vi "时间与数值的转换.vi"() -> ()   [LabVIEW 2020]
doc: "本VI是为《我和LabVIEW》一书编写的示例。\n关于本书的介绍请参考网页：\nhttp://ruanqizhen.spaces.live.com/blog/cns!5852D4F797C53FB6!4310.entry"
panel:
  out "时间标识":timestamp
  out "手工转换整数部分":u64
  out "手工转换小数部分":ext format="%#.6f"
  out "内部类型":cluster{u64, u64} {"?" format="%016x"; "?" format="%016x"}
  out "直接转换得到的秒数":dbl format="%.6f"
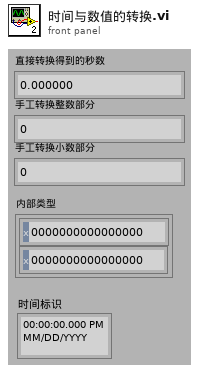
[diagram p1: front panel]
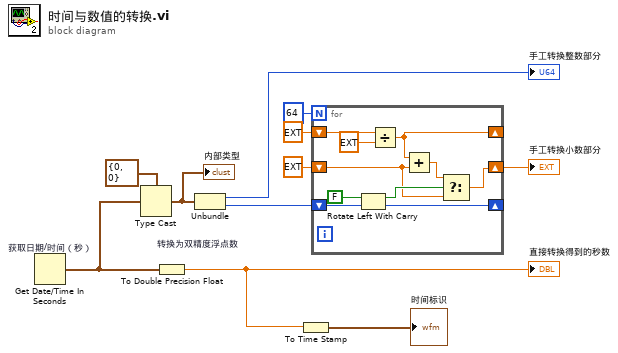
[diagram p0: block diagram]
diagram:
  n1 = Get Date/Time In Seconds "获取日期/时间（秒）"() -> (seconds since 1Jan1904=w11:timestamp)
  n2 = Type Cast(type=cluster{u64, u64} {0, 0}, x=w11) -> (*(type *) &x=w10:cluster{u64, u64})
  "内部类型" <- w10
  n3 = To Double Precision Float "转换为双精度浮点数"(number=w11) -> (double precision float=w2:dbl)
  "直接转换得到的秒数" <- w2
  n4 = Unbundle(w10) -> (→"手工转换整数部分":u64, w8:u64)
  n5 = To Time Stamp(1:w2) -> (0:→"时间标识":timestamp)
  n6 = for {
    N: 64 -> [_]
    shift-right: [w20] -> _
    shift-left: w8 -> [w21]
    shift-right: [w16] -> _
    shift-left: ext 1.0 -> [w19]
    shift-right: [w13] -> w6
    shift-left: ext 0.0 ("扩展精度浮点数") -> [w14]
    n7 = Rotate Left With Carry(2:w21, 3:FALSE ("进位")) -> (0:w20:u64, 1:w17:bool)
    n8 = Divide(x=w19, y=ext 2.0) -> (x/y=w16:ext)
    n9 = Add(x=w16, y=w14) -> (x+y=w15:ext)
    n10 = Select(t=w15, s=w17, f=w14) -> (s? t:f=w13:ext)
  }
  "手工转换小数部分" <- w6
